vi "ROI提取图像.vi"() -> ()   [LabVIEW 2018]
uses:
  <vilib>/vision/NI_Vision_Development_Module.lvlib
panel:
  out "error out":errorcluster
  out "Image 2":T1(plugin-control)
  out "Image":T1(plugin-control)
  in  "路径":path
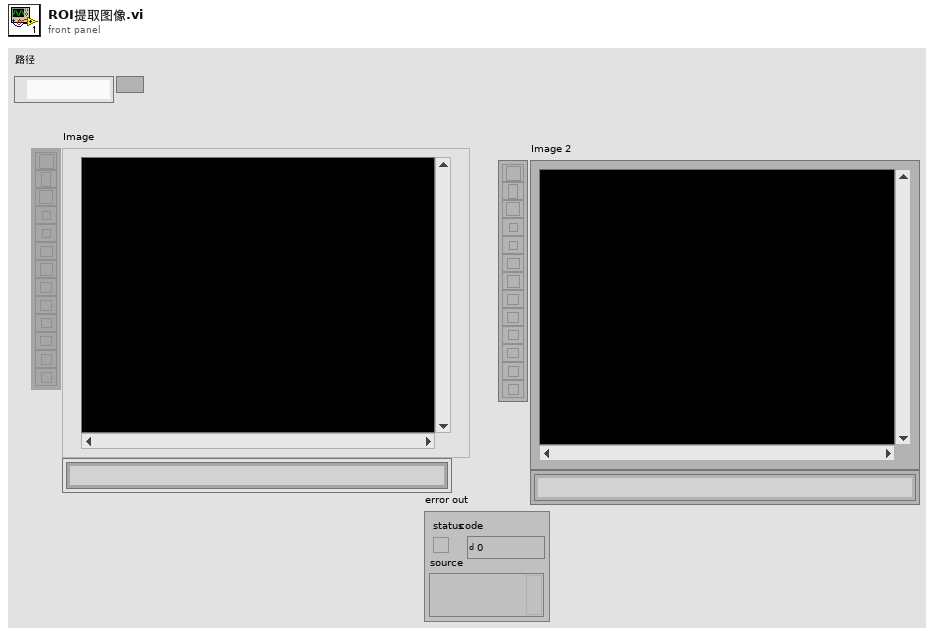
[diagram p1: front panel]
types:
  T1 = typedef "IMAQ Image.ctl" = refnum<image>
  T2 = typedef "IMAQ Rectangle" = cluster{"Left":i32, "Top":i32, "Right":i32, "Bottom":i32, "Rotation":dbl}
  T3 = typedef "ROI Descriptor" = cluster{"Global Rectangle":i32[], "Contours":cluster{"ID":enum32{"External", "Internal"}, "Type":u32, "Coordinates":i32[]}[]}
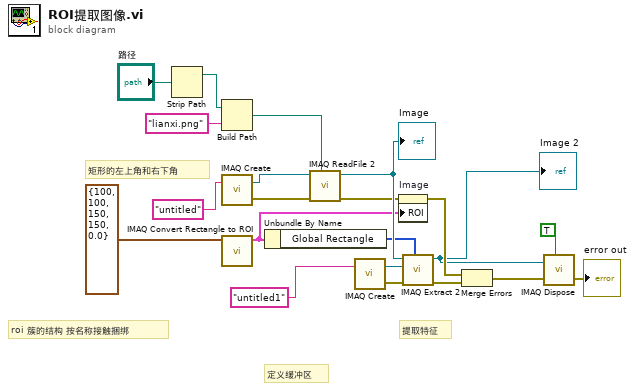
[diagram p0: block diagram]
diagram:
  # "矩形的左上角和右下角"
  # "roi 簇的结构 按名称接触捆绑"
  # "定义缓冲区"
  # "提取特征"
  n1 = Strip Path(path="路径") -> (stripped path=w20:path)  [unwired: 1 out]
  n2 = Build Path(base path=w20, name or relative path="lianxi.png" ("名称或相对路径")) -> (appended path=w15:path)
  n3 = call "IMAQ Create"("Image Name"="untitled") -> ("New Image"=w17:T1, "error out"=w16:errorcluster)  [unwired: 4 in]
  n4 = call "IMAQ Convert Rectangle to ROI"("Rectangle"=T2 {"Left"=100, "Top"=100, "Right"=150, "Bottom"=150, "Rotation"=0.0}) -> ("ROI Descriptor"=w9:T3)  [unwired: 8 in, 1 out]
  n5 = Unbundle By Name(w9) -> ("Global Rectangle"=w8:i32[])
  n6 = call "IMAQ ReadFile 2"("File Path"=w15, "error in (no error)"=w16, "Image"=w17) -> ("error out"=w7:errorcluster, "Image Out"=w10:T1)  [unwired: 4 in, 3 out]
  "Image" <- w10
  n7 = call "IMAQ Create"("Image Name"="untitled1") -> ("New Image"=w12:T1, "error out"=w11:errorcluster)  [unwired: 4 in]
  n8 = property on="Image" class="ImageControl"(error in=w7, "ROI"=w9) -> (error out=w5:errorcluster)  [unwired: 1 in, 1 out]
  n9 = call "IMAQ Extract 2"("Optional Rectangle"=w8, "error in (no error)"=w11, "Image Dst"=w12, "Image Src"=w10) -> ("error out"=w6:errorcluster, "Image Dst Out"=w3:T1)  [unwired: 6 in]
  "Image 2" <- w3
  n10 = Merge Errors(w5, w6) -> (w4:errorcluster)
  n11 = call "IMAQ Dispose"("All Images? (No)"=TRUE, "Image"=w3, "error in (no error)"=w4) -> ("error out"=→"error out":errorcluster)  [unwired: 3 in]
